vi "Vision_Right_R10.vi"() -> ()   [LabVIEW 2015]
uses:
  <vilib>/vision/Pattern Matching.llb/IMAQ Curve Parameters.ctl
  <vilib>/vision/Pattern Matching.llb/IMAQ Match Range Setting.ctl
panel:
  out "Right Image 2":T1(plugin-control)
  out "Frequency":sgl
  out "dT_ms":u32
  out "Avg Scale":dbl=84.09474029541016
  out "Avg Score":dbl=782.4534301757812
  out "Current Search Settings":T4={"Curve Parameters"={"Extraction Mode"=1, "Edge Threshold"=150, "Edge Filter Size"=0, "Min Length"=25, "Row Search Step Size"=15, "Col Search Step Size"=15, "Max Endpoint Gap"=2, "Closed"=TRUE, "Subpixel"=TRUE}, "Match Mode"={"Rotation"=TRUE, "Scale"=TRUE, "Occlusion"=FALSE, "Reserved"=FALSE, "Reserved"=FALSE, "Reserved"=FALSE}, "Range Settings"=[{"Match Constraints"=0, "Min"=-5.0, "Max"=5.0}, {"Match Constraints"=1, "Min"=79.09474029541016, "Max"=89.09474029541016}, {"Match Constraints"=2, "Min"=0.0, "Max"=0.0}], "Number of Matches"=1, "Minimum Match Score"=700.0, "SubPixel Accuracy"=TRUE, "Adv. Geometric Match Options 2"=[{"Setup Data Item"=20, "Item Value"=0.0}, {"Setup Data Item"=22, "Item Value"=1.0}]} {"Curve Parameters"."Extraction Mode" items=["Normal", "Uniform Regions"]; "Curve Parameters"."Edge Filter Size" items=["Fine", "Normal", "Contour Tracing"]; "Curve Parameters"."Max Endpoint Gap" min=0; "Curve Parameters"."Col Search Step Size" min=1 max=255 step=1; "Curve Parameters"."Row Search Step Size" min=1 max=255 step=1; "Curve Parameters"."Min Length" min=0; "Curve Parameters"."Edge Threshold" min=1 max=350 step=1; "Range Settings"."Max" format="%.2f"; "Range Settings"."Min" format="%.2f"; "Range Settings"."Match Constraints" items=["Rotation Angle (degrees)", "Scale Factor (%)", "Occlusion (%)"]}
  out "Valid Scale History":dbl[](array[numeric])=[84.05313110351562, 0.0, 84.23233795166016, 0.0, 84.0785140991211, 0.0, 84.0785140991211, 0.0, 84.03120422363281, 0.0, 84.09584045410156, 0.0, 84.12125396728516, 0.0, 84.0785140991211, 0.0, 84.0785140991211, 0.0, 84.0785140991211, 0.0] format="%#_13g"
  out "Valid Score History":dbl[](array[numeric])=[784.1742553710938, 0.0, 784.6376342773438, 0.0, 779.5546264648438, 0.0, 779.5546264648438, 0.0, 784.3460083007812, 0.0, 785.4644775390625, 0.0, 784.8938598632812, 0.0, 780.2630615234375, 0.0, 779.5546264648438, 0.0, 778.2620849609375, 0.0] format="%#_13g"
  out "Valid Beacon History - in":bool[](array[boolean])=[TRUE, FALSE, TRUE, FALSE, TRUE, FALSE, TRUE, FALSE, TRUE, FALSE, TRUE, FALSE, TRUE, FALSE, TRUE, FALSE, TRUE, FALSE, TRUE, FALSE]
  out "Startup Flag":bool
  out "Current Tempalte State":enum16{"Short Range", "Long Range"}(ring)
  out "Lock Status":bool=TRUE
  out "Y Coordinates":sgl[](array[numeric])=[0.0, 153.36156, 158.79634, 0.0, 0.0]
  out "X Coordinates":sgl[](array[numeric])=[0.0, 99.11854, 156.64487, 0.0, 0.0]
  out "Beacons Found":bool[](array[boolean])=[FALSE, TRUE, TRUE, FALSE, FALSE]
  in  "Initial State":enum16{"Short Range", "Long Range"}(ring)
  in  "History Size":i32=20
  in  "INITIAL Search Settings":T4={"Curve Parameters"={"Extraction Mode"=1, "Edge Threshold"=150, "Edge Filter Size"=0, "Min Length"=25, "Row Search Step Size"=15, "Col Search Step Size"=15, "Max Endpoint Gap"=2, "Closed"=TRUE, "Subpixel"=TRUE}, "Match Mode"={"Rotation"=TRUE, "Scale"=TRUE, "Occlusion"=TRUE, "Reserved"=FALSE, "Reserved"=FALSE, "Reserved"=FALSE}, "Range Settings"=[{"Match Constraints"=0, "Min"=-5.0, "Max"=5.0}, {"Match Constraints"=1, "Min"=20.0, "Max"=60.0}, {"Match Constraints"=2, "Min"=0.0, "Max"=25.0}], "Number of Matches"=1, "Minimum Match Score"=750.0, "SubPixel Accuracy"=TRUE, "Adv. Geometric Match Options 2"=[{"Setup Data Item"=20, "Item Value"=0.0}, {"Setup Data Item"=22, "Item Value"=1.0}]} {"Curve Parameters"."Extraction Mode" items=["Normal", "Uniform Regions"]; "Curve Parameters"."Edge Filter Size" items=["Fine", "Normal", "Contour Tracing"]; "Curve Parameters"."Max Endpoint Gap" min=0; "Curve Parameters"."Col Search Step Size" min=1 max=255 step=1; "Curve Parameters"."Row Search Step Size" min=1 max=255 step=1; "Curve Parameters"."Min Length" min=0; "Curve Parameters"."Edge Threshold" min=1 max=350 step=1; "Range Settings"."Max" format="%.2f"; "Range Settings"."Min" format="%.2f"; "Range Settings"."Match Constraints" items=["Rotation Angle (degrees)", "Scale Factor (%)", "Occlusion (%)"]; "Adv. Geometric Match Options 2"."Setup Data Item" items=["Curve Extraction Mode", "Curve Edge Threshold", "Curve Edge Filter Size", "Min Curve Length", "Curve Row Search Step Size", "Curve Col Search Step Size", "Curve Max Endpoint Gap", "Extract Closed Curves", "Enable Subpixel Curve Extraction", "Enable Correlation Score", "Enable Subpixel Accuracy", "Subpixel Iterations", "Subpixel Tolerance", "Initial Match List Length", "Enable Target Template Curve Score", "Min Match Separation Distance", "Min Match Separation Angle", "Min Match Separation Scale", "Max Match Overlap", "Enable Coarse Result", "Enable Calibration Support", "Enable Contrast Reversal", "Search Strategy", "Refinement Match Factor", "Subpixel Match Factor"]}
  # "Range"
  # "Range"
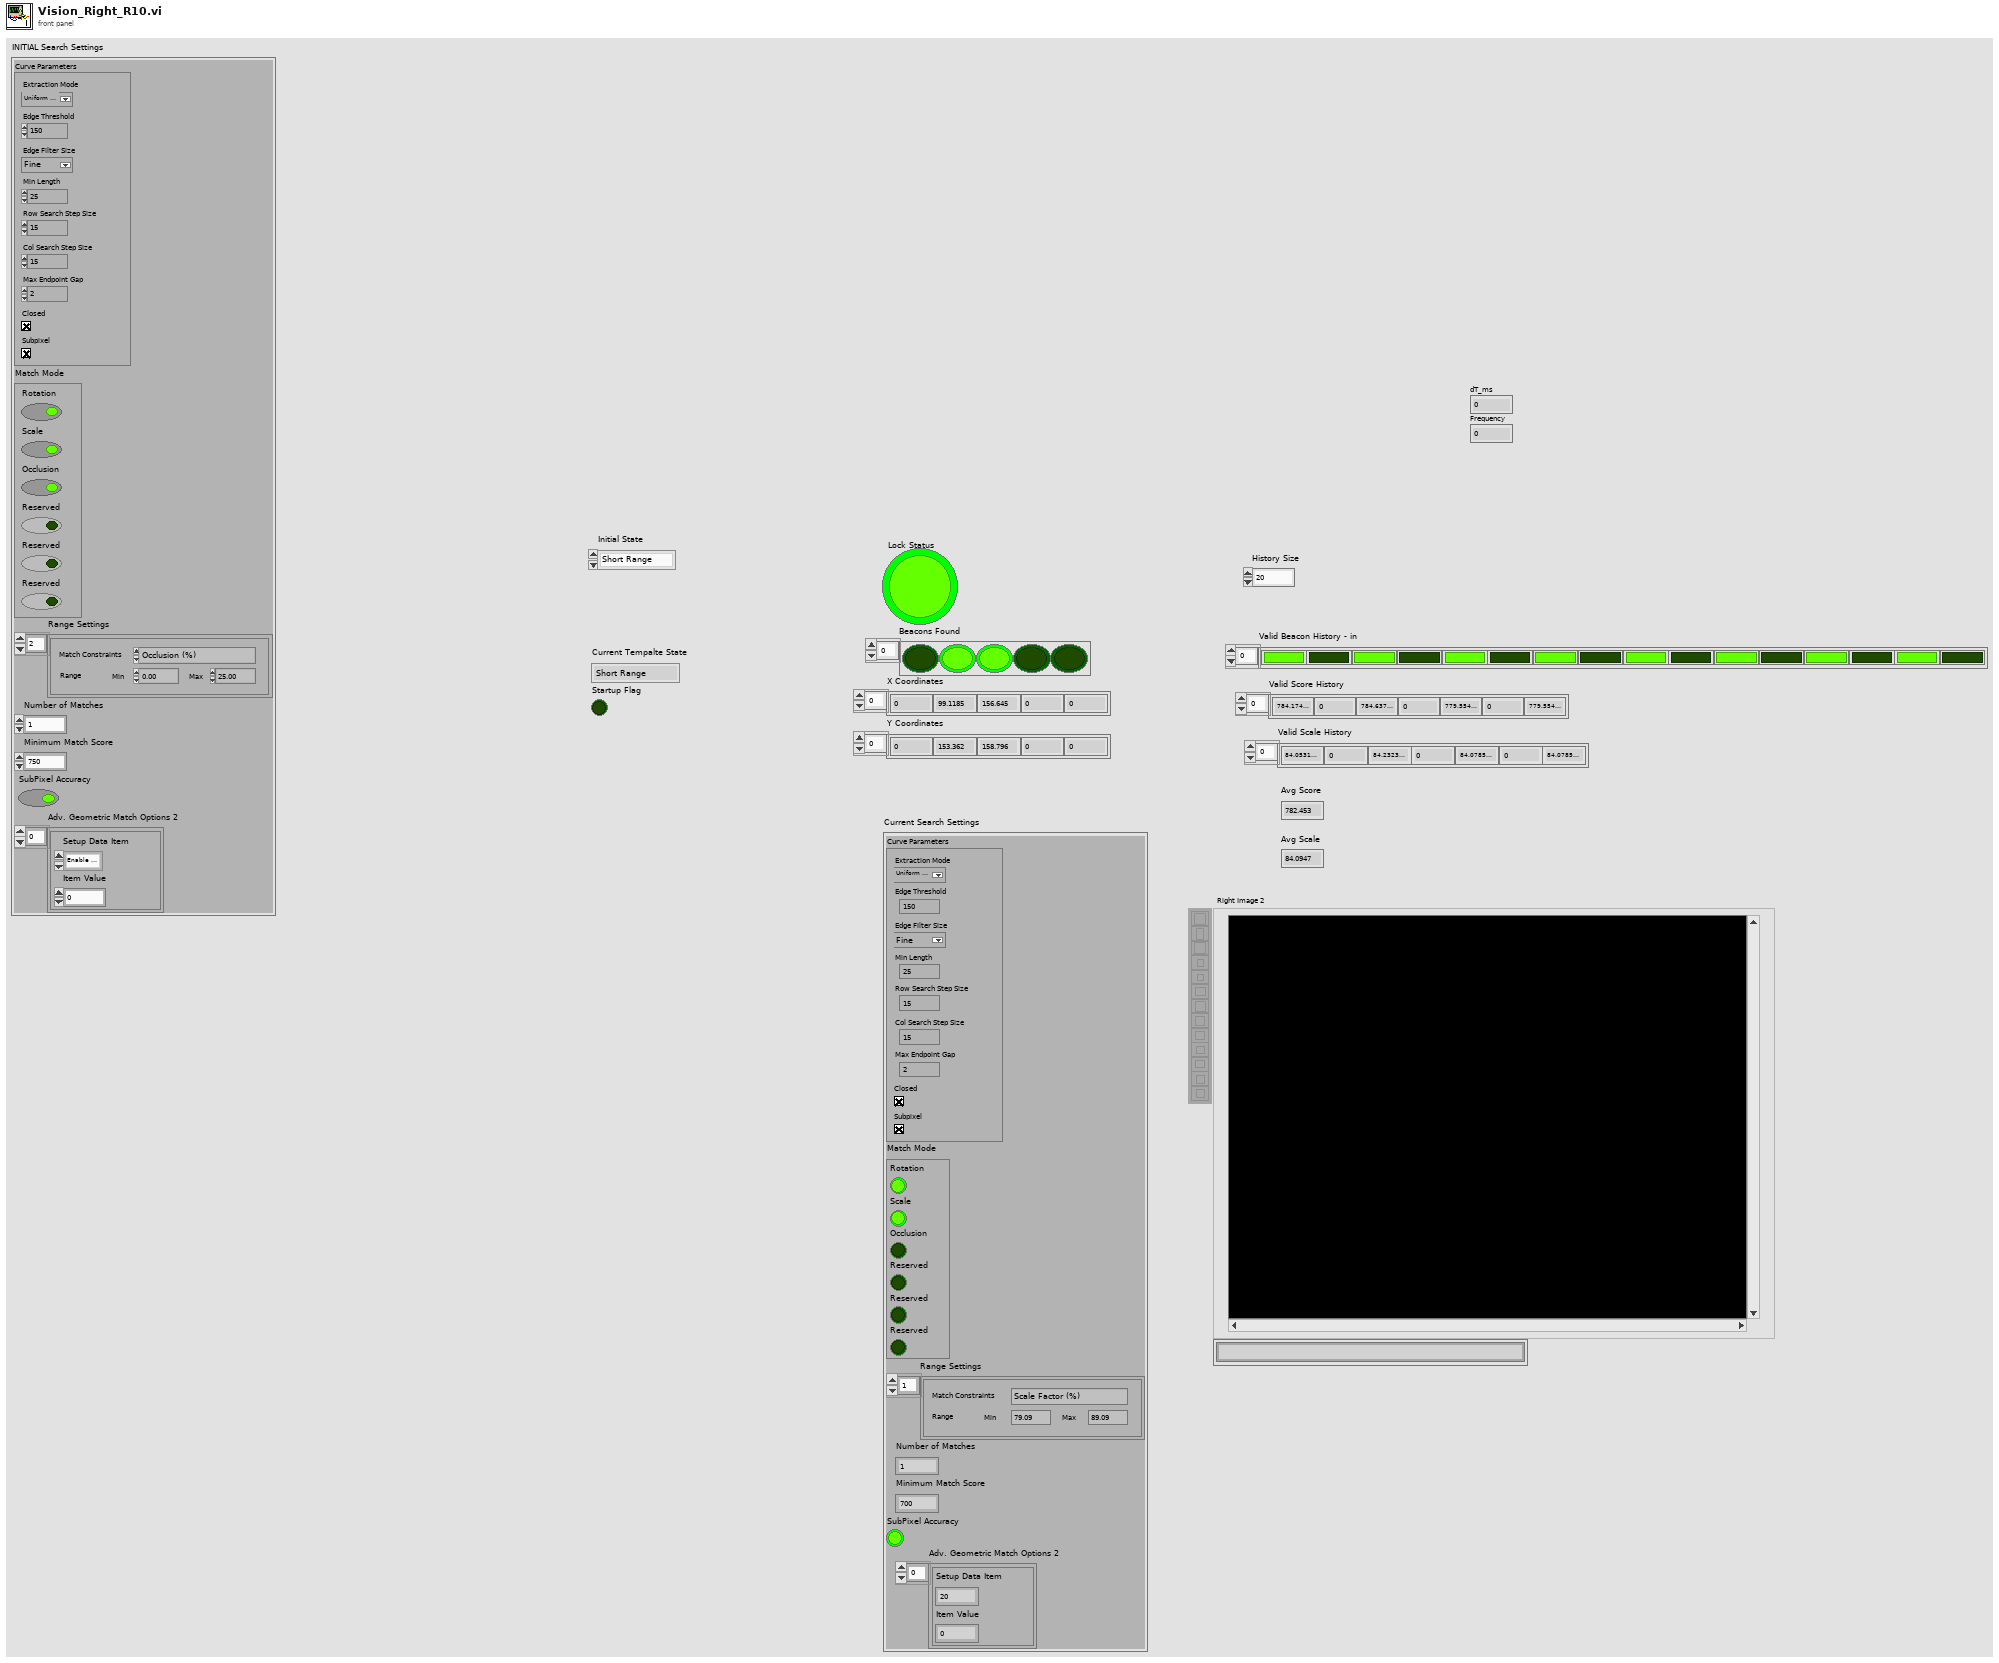
[diagram p1: front panel]
types:
  T1 = typedef "IMAQ Image.ctl" = refnum<image>
  T2 = typedef "IMAQ Curve Parameters.ctl" = cluster{"Extraction Mode":u32, "Edge Threshold":i32, "Edge Filter Size":u32, "Min Length":i32, "Row Search Step Size":i32, "Col Search Step Size":i32, "Max Endpoint Gap":i32, "Closed":bool, "Subpixel":bool}
  T3 = typedef "IMAQ Match Range Setting.ctl" = cluster{"Match Constraints":u32, "Min":dbl, "Max":dbl}
  T4 = cluster{"Curve Parameters":T2, "Match Mode":cluster{"Rotation":bool, "Scale":bool, "Occlusion":bool, "Reserved":bool, "Reserved":bool, "Reserved":bool}, "Range Settings":T3[], "Number of Matches":i32, "Minimum Match Score":sgl, "SubPixel Accuracy":bool, "Adv. Geometric Match Options 2":cluster{"Setup Data Item":u16, "Item Value":dbl}[]}
  T5 = typedef "Image Type" = u32
  T6 = typedef "ROI Descriptor" = cluster{"Global Rectangle":i32[], "Contours":cluster{"ID":enum32{"External", "Internal"}, "Type":u32, "Coordinates":i32[]}[]}
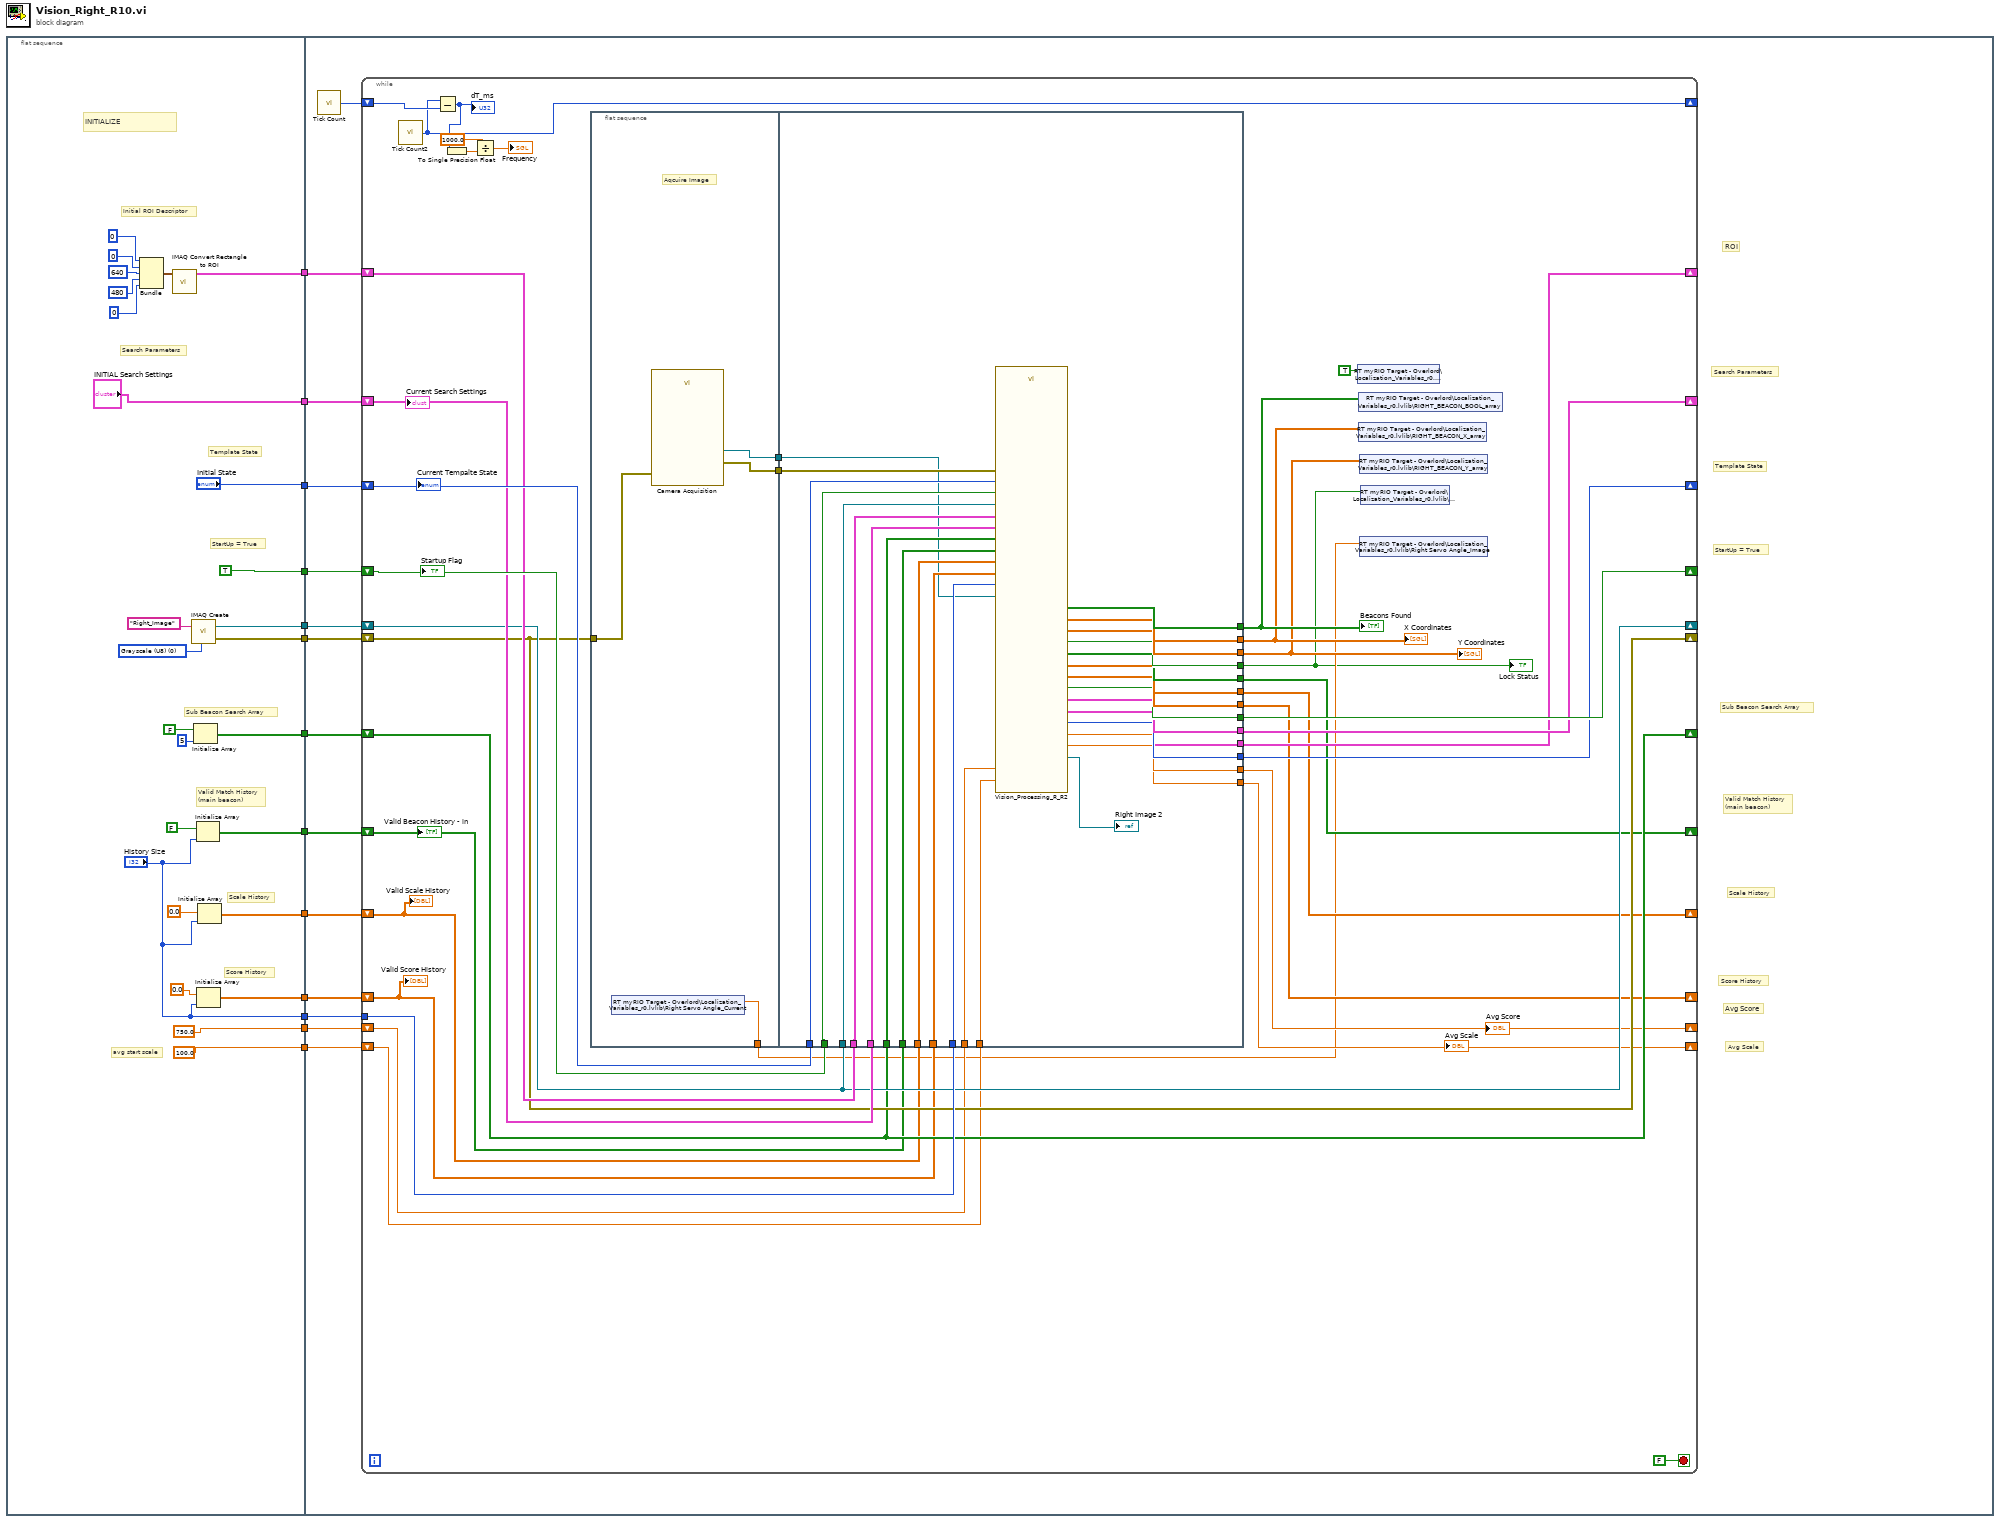
[diagram p0: block diagram]
diagram:
  n1 = flat-sequence {
    tunnel: [w26] -> w13
    tunnel: ["INITIAL Search Settings"] -> w12
    tunnel: ["Initial State"] -> w11
    tunnel: [TRUE] -> w10
    tunnel: [w23] -> w9
    tunnel: [w22] -> w8
    tunnel: [w21] -> w7
    tunnel: [w20] -> w6
    tunnel: [w19] -> w5
    tunnel: [w18] -> w4
    tunnel: ["History Size"] -> w3
    tunnel: [750.0] -> w2
    tunnel: [100.0] -> w1
    tunnel: w13 -> [w53]
    tunnel: w12 -> [w52]
    tunnel: w11 -> [w51]
    tunnel: w10 -> [w50]
    tunnel: w9 -> [w45]
    tunnel: w8 -> [w44]
    tunnel: w7 -> [w49]
    tunnel: w6 -> [w48]
    tunnel: w5 -> [w47]
    tunnel: w4 -> [w46]
    tunnel: w3 -> [w43]
    tunnel: w2 -> [w42]
    tunnel: w1 -> [w41]
    frame #0 {
      w33 = T5 0 items=["Grayscale (U8)", "Grayscale (I16)", "Grayscale (SGL)", "Complex (CSG)", "RGB (U32)", "HSL (U32)", "RGB (U64)", "Grayscale (U16)"] ("Image Type")
      # "avg start scale"
      # "Score History"
      # "Scale History"
      # "Valid Match History\n(main beacon)"
      # "Sub Beacon Search Array"
      # "Template State"
      # "Search Parameters"
      # "StartUp = True"
      # "Initial ROI Descriptor"
      # "INITIALIZE"
      n2 = Bundle(0, 0, 640, 480, 0) -> (w32:cluster{i32, i32, i32, i32, i32})  [unwired: 1 in]
      n3 = call "IMAQ Convert Rectangle to ROI"("Rectangle"=w32) -> ("ROI Descriptor"=w26:T6)  [unwired: 8 in, 1 out]
      n4 = call "IMAQ Create"("Image Name"="Right_Image", "Image Type"=w33) -> ("New Image"=w23:T1, "error out"=w22:errorcluster)  [unwired: 3 in]
      n5 = Initialize Array(FALSE, 5 ("dimension size")) -> (w21:bool[])
      n6 = Initialize Array(FALSE, "History Size") -> (w20:bool[])
      n7 = Initialize Array(0.0, "History Size") -> (w18:dbl[])
      n8 = Initialize Array(0.0, "History Size") -> (w19:dbl[])
    }
    frame #1 {
      # "Avg Scale"
      # "Avg Score"
      # "Score History"
      # "Scale History"
      # "Valid Match History\n(main beacon)"
      # "Sub Beacon Search Array"
      # "StartUp = True"
      # "Template State"
      # "Search Parameters"
      # "ROI"
      n9 = call "Tick Count"() -> ("Tick Count(mSec)"=w40:u32)
      n10 = while {
        shift-right: [w77] -> _
        shift-left: w53 -> [w85]
        shift-right: [w78] -> _
        shift-left: w52 -> [w84]
        shift-right: [w79] -> _
        shift-left: w51 -> [w88]
        shift-right: [w80] -> _
        shift-left: w50 -> [w86]
        shift-right: [w76] -> _
        shift-left: w49 -> [w76]
        shift-right: [w75] -> _
        shift-left: w48 -> [w72]
        shift-right: [w74] -> _
        shift-left: w47 -> [w71]
        shift-right: [w73] -> _
        shift-left: w46 -> [w70]
        shift-right: [w82] -> _
        shift-left: w45 -> [w82]
        shift-right: [w81] -> _
        shift-left: w44 -> [w81]
        tunnel: w43 -> [w83]
        shift-right: [w69] -> _
        shift-left: w42 -> [w67]
        shift-right: [w68] -> _
        shift-left: w41 -> [w66]
        shift-right: [w58] -> _
        shift-left: w40 -> [w59]
        stop <- FALSE stop-if-true
        n11 = call "Tick Count2"() -> ("Tick Count(mSec)"=w58:u32)
        n12 = Subtract(x=w58, y=w59) -> (x-y=w57:u32)
        "dT_ms" <- w57
        n13 = To Single Precision Float(number=w57) -> (single precision float=w56:sgl)
        n14 = Divide(x=sgl 1000.0, y=w56) -> (x/y=→"Frequency":sgl)
        n15 = flat-sequence {
          tunnel: w81 -> [w94]
          tunnel: [w93] -> w89
          tunnel: [w92] -> w87
          tunnel: [w91] -> w61
          tunnel: w89 -> [w100]
          tunnel: w88 -> [w121]
          tunnel: w87 -> [w122]
          tunnel: w86 -> [w120]
          tunnel: w82 -> [w119]
          tunnel: w85 -> [w118]
          tunnel: w84 -> [w117]
          tunnel: w76 -> [w116]
          tunnel: w72 -> [w115]
          tunnel: w71 -> [w114]
          tunnel: w70 -> [w113]
          tunnel: w83 -> [w112]
          tunnel: w67 -> [w97]
          tunnel: [w111] -> w64
          tunnel: [w110] -> w63
          tunnel: [w109] -> w62
          tunnel: [w108] -> w60
          tunnel: [w107] -> w75
          tunnel: [w106] -> w74
          tunnel: [w105] -> w73
          tunnel: [w104] -> w80
          tunnel: [w103] -> w78
          tunnel: [w101] -> w77
          tunnel: [w102] -> w79
          tunnel: [w99] -> w69
          tunnel: [w98] -> w68
          tunnel: w66 -> [w96]
          frame #0 {
            # "Aqcuire Image"
            n16 = shared-variable "RT myRIO Target - Overlord\\Localization_Variables_r0.lvlib\\Right Servo Angle_Current"() -> (w91:dbl)  [unwired: 1 in, 1 out]
            n17 = call "Camera Acquisition"("error in"=w94) -> ("Image Out"=w93:T1, "error out"=w92:errorcluster)  [unwired: 24 in, 1 out]
          }
          frame #1 {
            n18 = call "Vision_Processing_R_R2.vi"("Current State"=w121, "Image Dst"=w119, "Inpute Image"=w100, "Startup Flag"=w120, "Valid Beacon History - in"=w115, "Current ROI Descriptor"=w118, "Avg Score - Last"=w97, "error in (no error)"=w122, "Current Settings"=w117, "Sub Beacon Search Enable"=w116, "Avg Scale - Last"=w96, "Valid Score History"=w113, "Valid Scale History"=w114, "History Size"=w112) -> ("Valid Scale History\nOut"=w106:dbl[], "Avg Scale"=w98:dbl, "Avg Score"=w99:dbl, "Valid Score History\nOut"=w105:dbl[], "Valid Beacon History\nOut"=w107:bool[], "Y Coordinates"=w109:sgl[], "Beacons Found"=w111:bool[], "X Coordinates"=w110:sgl[], "Next Main ROI Descriptor"=w101:T6, "Lock Status"=w108:bool, "Startup Flag - out"=w104:bool, "New Settings"=w103:T4, "Next State"=w102:enum16{"Short Range", "Long Range"}, "Right Image 2"=→"Right Image 2":T1)
          }
        }
        n19 = shared-variable "RT myRIO Target - Overlord\\Localization_Variables_r0.lvlib\\RIGHT_FLAG"(TRUE ("RIGHT_FLAG")) -> ()  [unwired: 1 in, 1 out]
        n20 = shared-variable "RT myRIO Target - Overlord\\Localization_Variables_r0.lvlib\\RIGHT_BEACON_BOOL_array"(w64) -> ()  [unwired: 1 in, 1 out]
        n21 = shared-variable "RT myRIO Target - Overlord\\Localization_Variables_r0.lvlib\\RIGHT_BEACON_X_array"(w63) -> ()  [unwired: 1 in, 1 out]
        n22 = shared-variable "RT myRIO Target - Overlord\\Localization_Variables_r0.lvlib\\RIGHT_BEACON_Y_array"(w62) -> ()  [unwired: 1 in, 1 out]
        n23 = shared-variable "RT myRIO Target - Overlord\\Localization_Variables_r0.lvlib\\Right Servo Angle_Image"(w61) -> ()  [unwired: 1 in, 1 out]
        n24 = shared-variable "RT myRIO Target - Overlord\\Localization_Variables_r0.lvlib\\Image Lock - R"(w60) -> ()  [unwired: 1 in, 1 out]
        "Beacons Found" <- w64
        "X Coordinates" <- w63
        "Y Coordinates" <- w62
        "Lock Status" <- w60
        "Current Tempalte State" <- w88
        "Startup Flag" <- w86
        "Valid Scale History" <- w71
        "Valid Beacon History - in" <- w72
        "Valid Score History" <- w70
        "Current Search Settings" <- w84
        "Avg Score" <- w69
        "Avg Scale" <- w68
      }
    }
  }
